vi "Get Rx Monitor Error.vi"() -> (3 "Channel Array":string[](array[string]))   [LabVIEW 2020, in "AIM ARINC 664 GUID Utility.lvlib"]
uses:
  Scripting/Constants.vi
  AIM ARINC 664 GUID Utility.lvlib
  Scripting/AIM ARINC 664 Scripting.lvlib
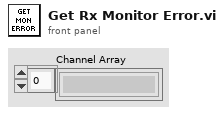
[diagram p1: front panel]
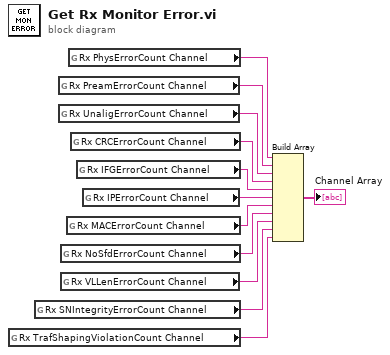
[diagram p0: block diagram]
diagram:
  n1 = global read "Constants.vi" "Rx TrafShapingViolationCount Channel"() -> (w2:string)
  n2 = global read "Constants.vi" "Rx SNIntegrityErrorCount Channel"() -> (w3:string)
  n3 = global read "Constants.vi" "Rx PreamErrorCount Channel"() -> (w11:string)
  n4 = global read "Constants.vi" "Rx UnaligErrorCount Channel"() -> (w10:string)
  n5 = global read "Constants.vi" "Rx NoSfdErrorCount Channel"() -> (w5:string)
  n6 = global read "Constants.vi" "Rx VLLenErrorCount Channel"() -> (w4:string)
  n7 = global read "Constants.vi" "Rx MACErrorCount Channel"() -> (w6:string)
  n8 = global read "Constants.vi" "Rx PhysErrorCount Channel"() -> (w12:string)
  n9 = global read "Constants.vi" "Rx CRCErrorCount Channel"() -> (w9:string)
  n10 = global read "Constants.vi" "Rx IFGErrorCount Channel"() -> (w8:string)
  n11 = global read "Constants.vi" "Rx IPErrorCount Channel"() -> (w7:string)
  n12 = Build Array(w12, w11, w10, w9, w8, w7, w6, w5, w4, w3, w2) -> (→"Channel Array":string[])
